vi "Robot Movement Command Interpreter - to robot.vi"(11 "Rubix Cmd":T1={"Rotate command"=enum."Middle row left", "Facet to act on"=0}) -> (3 "Rbt Cmd":string)   [LabVIEW 2019]
uses:
  facet and command.ctl
  Cube Data Ops.ctl
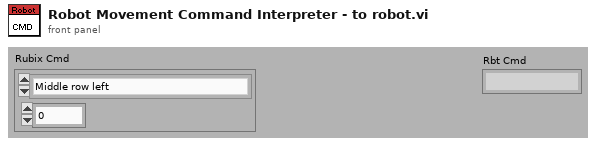
[diagram p1: front panel]
types:
  T1 = typedef "facet and command.ctl" = cluster{"Rotate command":T2, "Facet to act on":u8}
  T2 = typedef "Cube Data Ops.ctl" = enum16{"Initialize", "Set Rubix Ref Array", "Set Rubix Text Array", "Set Current Face", "Get Rubix Text Array", "Generate Rubix Array", "Get Rubix array", "Get Facets to move", "Randomize", "Top row left", "Top row right", "Middle row left", "Middle row right", "Bottom row left", "Bottom row right", "Left column up", "Left column down", "Middle column up", "Middle column down", "Right column up", "Right column down", "Face ccw", "Face cw"}
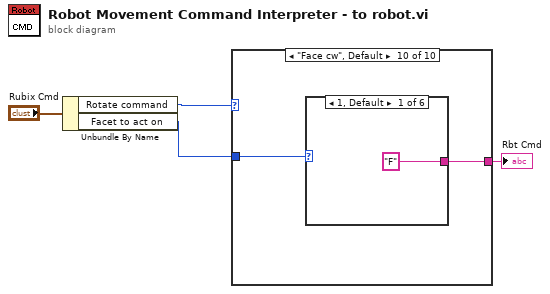
[diagram p0: block diagram]
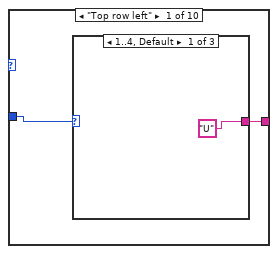
[diagram p2: hidden frame]
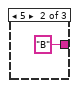
[diagram p3: hidden frame]
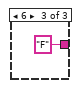
[diagram p4: hidden frame]
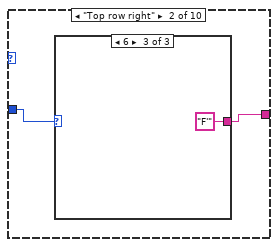
[diagram p5: hidden frame]
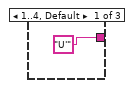
[diagram p6: hidden frame]
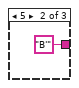
[diagram p7: hidden frame]
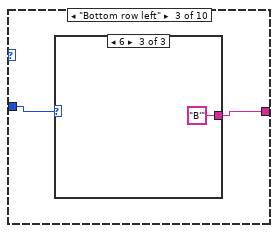
[diagram p8: hidden frame]
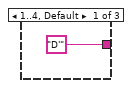
[diagram p9: hidden frame]
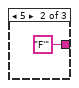
[diagram p10: hidden frame]
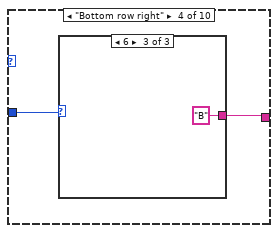
[diagram p11: hidden frame]
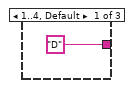
[diagram p12: hidden frame]
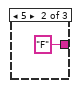
[diagram p13: hidden frame]
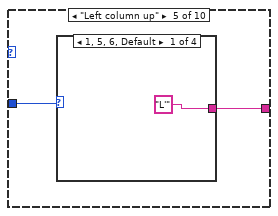
[diagram p14: hidden frame]
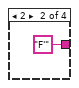
[diagram p15: hidden frame]
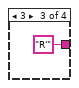
[diagram p16: hidden frame]
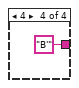
[diagram p17: hidden frame]
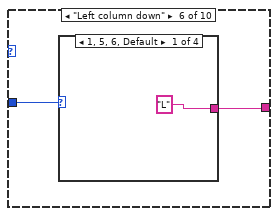
[diagram p18: hidden frame]
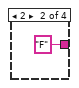
[diagram p19: hidden frame]
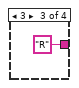
[diagram p20: hidden frame]
diagram:
  n1 = Unbundle By Name("Rubix Cmd") -> ("Rotate command"=w3:T2, "Facet to act on"=w2:u8)
  n2 = case shown="\"Face cw\", Default" w3 {
    tunnel: w2 -> [w5 w10 w15 w20 w25 w31 w38 w44 w50 w57]
    tunnel: [w6 w11 w16 w21 w26 w32 w37 w43 w49 w58] -> w1
    frame "Top row left" {
      n3 = case shown="1..4, Default" w5 {
        tunnel: ["U" "B" "F"] -> w6
        frame 1..4, Default {
        }
        frame 5 {
        }
        frame 6 {
        }
      }
    }
    frame "Top row right" {
      n4 = case shown="6" w10 {
        tunnel: ["U'" "B'" "F'"] -> w11
        frame 1..4, Default {
        }
        frame 5 {
        }
        frame 6 {
        }
      }
    }
    frame "Bottom row left" {
      n5 = case shown="6" w15 {
        tunnel: ["D'" "F'" "B'"] -> w16
        frame 1..4, Default {
        }
        frame 5 {
        }
        frame 6 {
        }
      }
    }
    frame "Bottom row right" {
      n6 = case shown="6" w20 {
        tunnel: ["D" "F" "B"] -> w21
        frame 1..4, Default {
        }
        frame 5 {
        }
        frame 6 {
        }
      }
    }
    frame "Left column up" {
      n7 = case shown="1, 5, 6, Default" w25 {
        tunnel: ["L'" "F'" "R'" "B'"] -> w26
        frame 1, 5, 6, Default {
        }
        frame 2 {
        }
        frame 3 {
        }
        frame 4 {
        }
      }
    }
    frame "Left column down" {
      n8 = case shown="1, 5, 6, Default" w31 {
        tunnel: ["L" "F" "R" "B"] -> w32
        frame 1, 5, 6, Default {
        }
        frame 2 {
        }
        frame 3 {
        }
        frame 4 {
        }
      }
    }
    frame "Right column up" {
      n9 = case shown="1, 5, 6, Default" w38 {
        tunnel: ["B" "F" "R" "L"] -> w37
        frame 2 {
        }
        frame 4 {
        }
        frame 1, 5, 6, Default {
        }
        frame 3 {
        }
      }
    }
    frame "Right column down" {
      n10 = case shown="4" w44 {
        tunnel: ["B'" "F'" "R'" "L'"] -> w43
        frame 2 {
        }
        frame 4 {
        }
        frame 1, 5, 6, Default {
        }
        frame 3 {
        }
      }
    }
    frame "Face ccw" {
      n11 = case shown="6" w50 {
        tunnel: ["F'" "R'" "B'" "L'" "U'" "D'"] -> w49
        frame 1, Default {
        }
        frame 2 {
        }
        frame 3 {
        }
        frame 4 {
        }
        frame 5 {
        }
        frame 6 {
        }
      }
    }
    frame "Face cw", Default {
      n12 = case shown="1, Default" w57 {
        tunnel: ["F" "R" "B" "L" "U" "D"] -> w58
        frame 1, Default {
        }
        frame 2 {
        }
        frame 3 {
        }
        frame 4 {
        }
        frame 5 {
        }
        frame 6 {
        }
      }
    }
  }
  "Rbt Cmd" <- w1
